vi "Globals.vi"() -> ()   [LabVIEW 2016]
panel:
  in  "loader state":i32
  in  "VisionOverlayIndex":dbl
  in  "Pitch tireur":dbl(knob) scale=-1.0..1.0
  out "Feed me":bool
  out "Step moter steps":dbl
  in  "Absolute Distance (inches)":dbl
  in  "Distance (inches)":dbl
  out "Sensor Droite (inches)":dbl
  out "Sensor Gauche (inches)":dbl
  # "Telemetry"
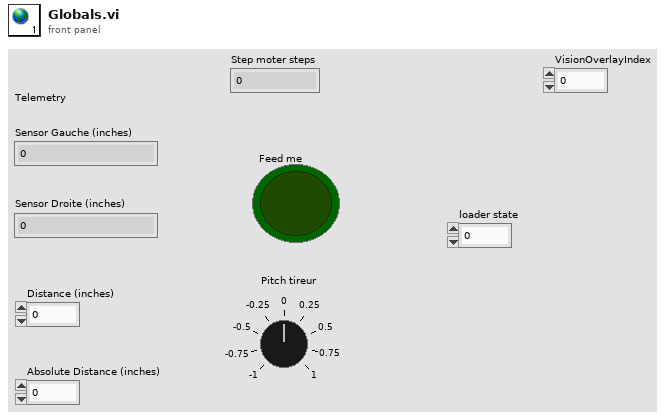
[diagram p1: front panel]
diagram:
